vi "Evaluate.vi"(8 "error in (no error)":errorcluster, 11 "One or More In":refnum<class "At Least.lvclass">) -> (0 "error out":errorcluster, 1 "Message":string, 2 "Passed?":bool)   [LabVIEW 2020, in "Deprecated At Least.lvlib" / "At Least.lvclass"]
uses:
  At Least.lvclass
  At Least.lvclass/At Least.ctl
  Core/VI Call/VI Call.lvclass
  Core/Comparator/Comparator.lvclass
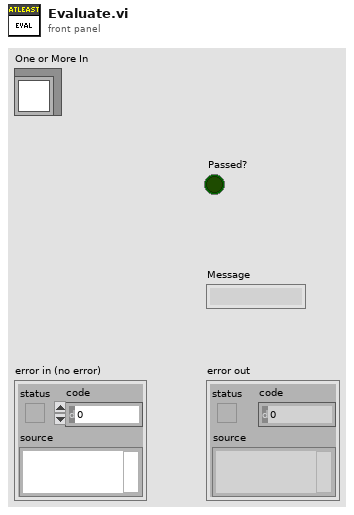
[diagram p1: front panel]
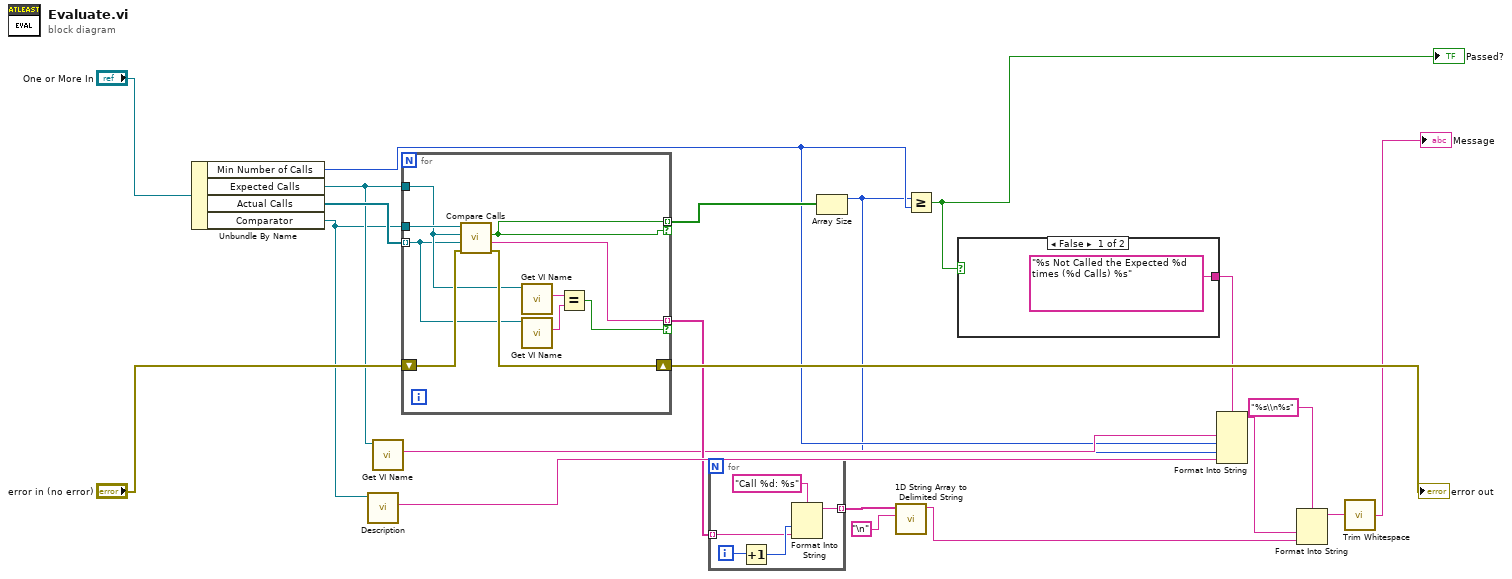
[diagram p0: block diagram]
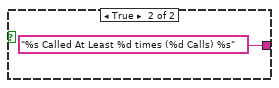
[diagram p2: hidden frame]
diagram:
  n1 = Unbundle By Name("One or More In") -> ("Min Number of Calls"=w3:i32, "Expected Calls"=w15:refnum<class "VI Call.lvclass">, "Actual Calls"=w19:refnum<class "VI Call.lvclass">[], "Comparator"=w14:refnum<class "Comparator.lvclass">)
  n2 = call-dynamic "Description.vi"("Comparator in"=w14) -> ("Description"=w16:string)  [unwired: 9 in, 1 out]
  n3 = call-dynamic "Get VI Name.vi"("VI Call In"=w15) -> ("VI Name"=w4:string)  [unwired: 10 in]
  n4 = for {
    tunnel: w15 -> [w23]
    tunnel: w14 -> [w31]
    tunnel: w19 -> [w22] mode=indexing
    shift-right: [w29] -> w17
    shift-left: "error in (no error)" -> [w30]
    tunnel: [w28] -> w20 mode=indexing if=w28
    tunnel: [w27] -> w5 mode=indexing if=w24
    n5 = call-dynamic "Compare Calls.vi"("error in (no error)"=w30, "VI Call 2"=w22, "VI Call 1"=w23, "Comparator in"=w31) -> ("error out"=w29:errorcluster, "Description"=w27:string, "Equal?"=w28:bool)  [unwired: 5 in]
    n6 = call-dynamic "Get VI Name.vi"("VI Call In"=w23) -> ("VI Name"=w26:string)  [unwired: 10 in]
    n7 = call-dynamic "Get VI Name.vi"("VI Call In"=w22) -> ("VI Name"=w25:string)  [unwired: 10 in]
    n8 = Equal?(x=w26, y=w25) -> (x = y?=w24:bool)
  }
  "error out" <- w17
  n9 = for {
    tunnel: w5 -> [w33] mode=indexing
    tunnel: [w32] -> w6 mode=indexing
    i -> [w35]
    n10 = Increment(x=w35) -> (x+1=w34:i32)
    n11 = Format Into String(format string="Call %d: %s", w34, w33) -> (resulting string=w32:string)  [unwired: 2 in, 1 out]
  }
  n12 = Array Size(array=w20) -> (size(s)=w2:i32)
  n13 = call <vilib>:"1D String Array to Delimited String.vi"("delimiter"="\n", "string array"=w6) -> ("delimited string"=w8:string)  [unwired: 9 in]
  n14 = Greater Or Equal?(x=w2, y=w3) -> (x >= y?=w1:bool)
  "Passed?" <- w1
  n15 = case shown="False" w1 {
    tunnel: ["%s Not Called the Expected %d times (%d Calls) %s" ("Message") "%s Called At Least %d times (%d Calls) %s" ("Message")] -> w13
    frame False {
    }
    frame True {
    }
  }
  n16 = Format Into String(format string=w13, w4, w3, w2, w16) -> (resulting string=w7:string)  [unwired: 2 in, 1 out]
  n17 = Format Into String(format string="%s\\n%s", w7, w8) -> (resulting string=w11:string)  [unwired: 2 in, 1 out]
  n18 = call <vilib>:"Trim Whitespace.vi"("string"=w11) -> ("trimmed string"=→"Message":string)  [unwired: 1 in]
